vi "Replace Or Add Robots.vi"(10 "Robots New":T1[](array[typedef]) {"height" format="%+4.3f"; "pixel_y" format="%+4.3f"; "pixel_x" format="%+4.3f"; "orientation" format="%+4.3f"; "y" format="%+4.3f"; "confidence" format="%4.3f"; "x" format="%+4.3f"}, 11 "Robots Old":T1[](array[typedef]) {"height" format="%+4.3f"; "pixel_y" format="%+4.3f"; "pixel_x" format="%+4.3f"; "orientation" format="%+4.3f"; "y" format="%+4.3f"; "confidence" format="%4.3f"; "x" format="%+4.3f"}) -> (3 "Robots New Out":T1[](array[typedef]) {"height" format="%+4.3f"; "pixel_y" format="%+4.3f"; "pixel_x" format="%+4.3f"; "orientation" format="%+4.3f"; "y" format="%+4.3f"; "confidence" format="%4.3f"; "x" format="%+4.3f"})   [LabVIEW 2016]
uses:
  SSL Detection Robot.ctl
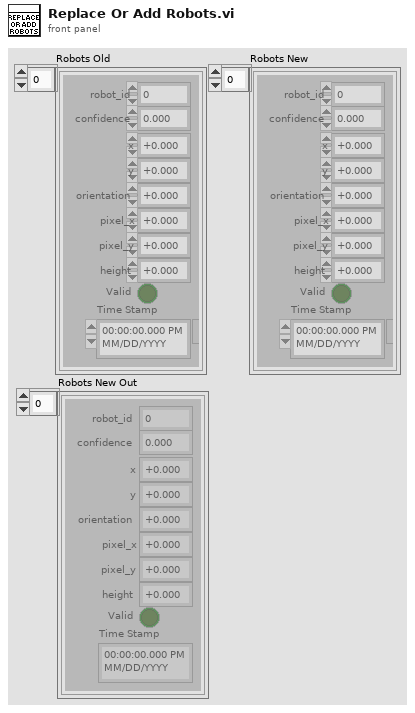
[diagram p1: front panel]
types:
  T1 = typedef "SSL Detection Robot.ctl" = cluster{"x":sgl, "robot_id":u32, "confidence":sgl, "y":sgl, "orientation":sgl, "pixel_x":sgl, "pixel_y":sgl, "height":sgl, "Valid":bool, "Time Stamp":timestamp}
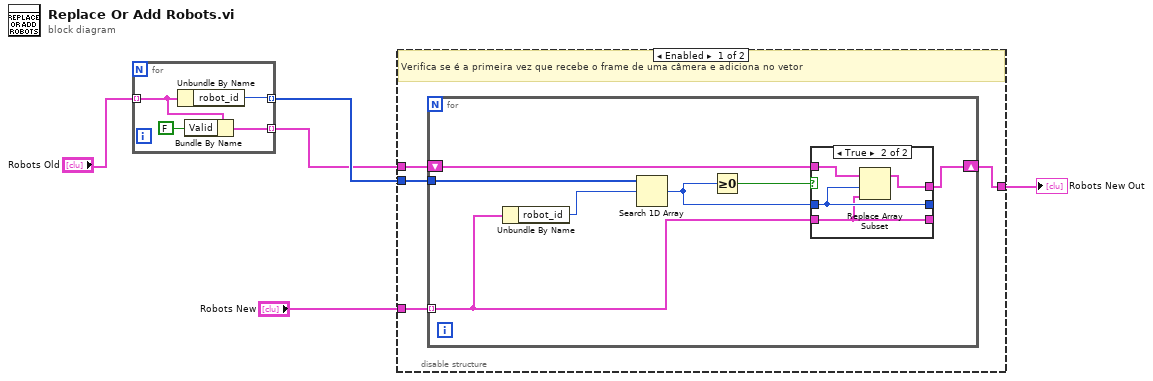
[diagram p0: block diagram]
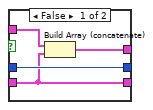
[diagram p2: hidden frame]
diagram:
  n1 = for {
    tunnel: "Robots Old" -> [w8] mode=indexing
    tunnel: [w9] -> w3 mode=indexing
    tunnel: [w6] -> w1 mode=indexing
    n2 = Unbundle By Name(w8) -> ("robot_id"=w9:u32)
    n3 = Bundle By Name(cluster=w8, "Valid"=FALSE) -> (w6:T1)
  }
  n4 = disable-structure "Diagram Disable Structure" shown="Enabled" {
    disable-tunnel: w1 -> [w13 _]
    disable-tunnel: "Robots New" -> [w12 _]
    disable-tunnel: [w11 _] -> w4
    disable-tunnel: w3 -> [w10 _]
    frame Enabled {
      # "Verifica se é a primeira vez que recebe o frame de uma câmera e adiciona no vetor"
      n5 = for {
        tunnel: w12 -> [w17] mode=indexing
        tunnel: w10 -> [w18]
        shift-right: [w19] -> w11
        shift-left: w13 -> [w20]
        n6 = Unbundle By Name(w17) -> ("robot_id"=w16:u32)
        n7 = Search 1D Array(1D array=w18, element=w16) -> (index of element=w14:i32)  [unwired: 1 in]
        n8 = Greater Or Equal To 0?(x=w14) -> (x >= 0?=w15:bool)
        n9 = case shown="True" w15 {
          tunnel: w20 -> [w24 w28]
          tunnel: w17 -> [w21 w26]
          tunnel: [w23 w25] -> w19
          tunnel: w14 -> [w22 w27]
          tunnel: [w22 w27] -> _
          tunnel: [w21 w26] -> _
          frame False {
            n10 = Build Array (concatenate)(w24, w21) -> (w23:T1[])
          }
          frame True {
            n11 = Replace Array Subset(array=w28, new element=w26, index=w27) -> (w25:T1[])
          }
        }
      }
    }
    frame Disabled {
    }
  }
  "Robots New Out" <- w4
